vi "Mark_GetBEMark.vi"(6 "Type (Time)":enum16{"Time", "Percentage", "Index"}(ring), 8 "error in (no error)":errorcluster, 11 "ExpData In":refnum<class "ExpData.lvclass">) -> (0 "error out":errorcluster, 1 "End":dbl[](array[numeric]), 2 "Begin":dbl[](array[numeric]), 3 "ExpData Out":refnum<class "ExpData.lvclass">, 4 "Total Length":i32)   [LabVIEW 2015, in "ExpData.lvclass"]
uses:
  ExpData.lvclass
  ExpData.lvclass/ExpData.ctl
  <userlib>/_OpenG.lib/array/array.llb/Index 1D Array Elements (DBL)__ogtk.vi
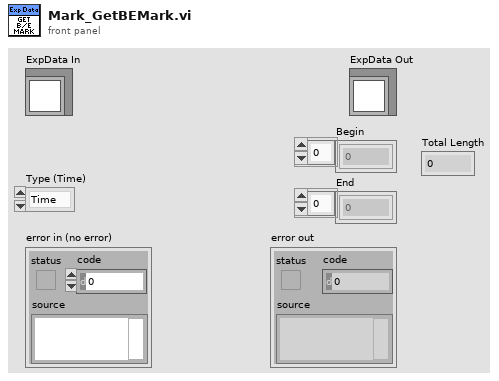
[diagram p1: front panel]
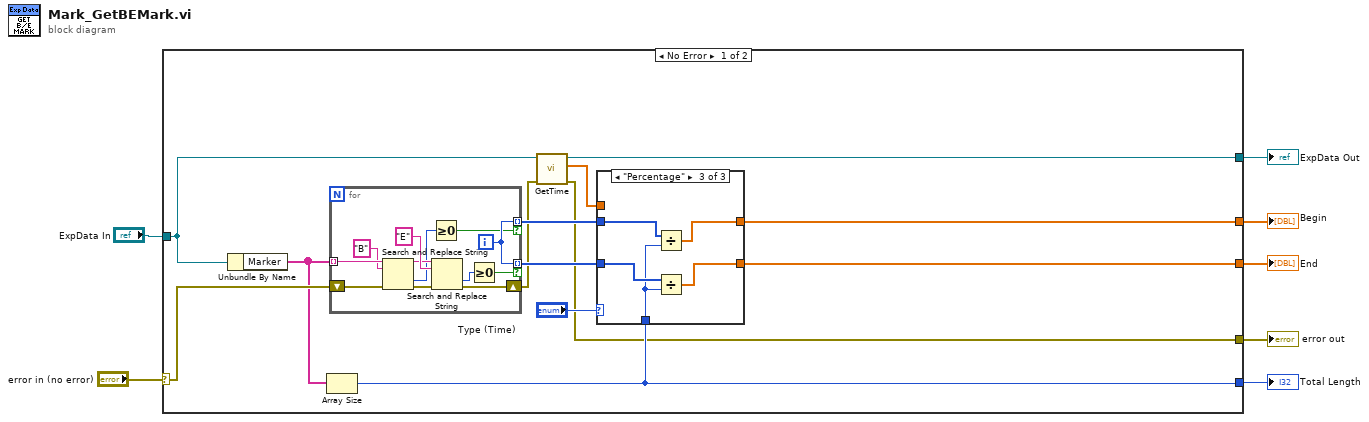
[diagram p0: block diagram]
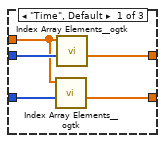
[diagram p2: hidden frame]
diagram:
  n1 = case shown="No Error" "error in (no error)" {
    selector: "error in (no error)" -> [w20 w48]
    tunnel: [w10 w48] -> w7
    tunnel: "ExpData In" -> [w14 w45]
    tunnel: [w9 i32[] []] -> w4
    tunnel: [w8 i32[] []] -> w3
    tunnel: [w13 w45] -> w2
    tunnel: [w16 _] -> w1
    frame No Error {
      n2 = Unbundle By Name(w14) -> ("Marker"=w19:string[])
      n3 = Array Size(array=w19) -> (size(s)=w16:i32)
      n4 = for {
        tunnel: w19 -> [w44] mode=indexing
        shift-right: [w38] -> w11
        shift-left: w20 -> [w43]
        tunnel: [w34] -> w18 mode=indexing if=w35
        tunnel: [w34] -> w17 mode=indexing if=w33
        i -> [w34]
        n5 = Search and Replace String(input string=w44, search string="B", error in=w43) -> (result string=w40:string, offset past replacement=w36:i32, error out=w39:errorcluster)  [unwired: 5 in, 1 out]
        n6 = Greater Or Equal To 0?(x=w36) -> (x >= 0?=w33:bool)
        n7 = Search and Replace String(input string=w40, search string="E", error in=w39) -> (offset past replacement=w37:i32, error out=w38:errorcluster)  [unwired: 5 in, 2 out]
        n8 = Greater Or Equal To 0?(x=w37) -> (x >= 0?=w35:bool)
      }
      n9 = call "GetTime.vi"("error in (no error)"=w11, "CarexMData in"=w14) -> ("error out"=w10:errorcluster, "Time"=w15:dbl[], "CarexMData out"=w13:refnum<class "ExpData.lvclass">)  [unwired: 7 in]
      n10 = case shown="\"Percentage\"" "Type (Time)" {
        tunnel: [w22 w26 w29] -> w8
        tunnel: w18 -> [w24 w26 w31]
        tunnel: [w21 w27 w28] -> w9
        tunnel: w17 -> [w25 w27 w32]
        tunnel: w16 -> [_ _ w30]
        tunnel: w15 -> [w23 _ _]
        frame "Time", Default {
          n11 = call-poly <userlib>:"Index Array Elements__ogtk.vi"("indices"=w24, "array"=w23) -> ("elements"=w22:dbl[])  [unwired: 9 in]
          n12 = call-poly <userlib>:"Index Array Elements__ogtk.vi"("indices"=w25, "array"=w23) -> ("elements"=w21:dbl[])  [unwired: 9 in]
        }
        frame "Index" {
        }
        frame "Percentage" {
          n13 = Divide(x=w32, y=w30) -> (x/y=w28:dbl[])
          n14 = Divide(x=w31, y=w30) -> (x/y=w29:dbl[])
        }
      }
    }
    frame Error {
    }
  }
  "ExpData Out" <- w2
  "error out" <- w7
  "Begin" <- w4
  "End" <- w3
  "Total Length" <- w1
